vi "日志报警状态存储 (子VI).vi"() -> ()   [LabVIEW 2016, in "斯坦道CODMn.lvlib"]
uses:
  <vilib>/ptbypt/NI_PtbyPt.lvlib
  <vilib>/Utility/config.llb/NI_LVConfig.lvlib
panel:
  out "多列列表框":i32(listbox)
  out "CODMn工作状态":T1(ring)
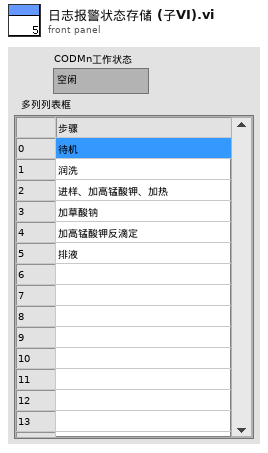
[diagram p1: front panel]
types:
  T1 = enum16{"空闲", "水样测试", "标样核查", "零点核查", "跨度核查", "空白测试", "平行样测试", "质控样", "空白校准", "标样校准", "加标回收"}
  T2 = cluster{"时间标识":timestamp, "设备":string, "日志信息":string}
  T3 = cluster{"时间标识":timestamp, "参数":string, "日志信息":string, "流程参数":string}
  T4 = cluster{"ORP故障":bool, "温控器故障":bool, "加热故障":bool, "高锰酸钾报警":bool, "草酸钠报警":bool, "测量错误":bool, "校零错误":bool, "校标错误":bool, " 进水样超量程":bool, "排液阀故障":bool, "60分钟超时报警":bool, "进样无液体报警":bool}
  T5 = cluster{"时间标识":timestamp, "设备":string, "日志信息":string, "流程参数":string}
  T6 = cluster{"测量量程":dbl, "测量精度":dbl, "测量间隔":dbl, "消解温度":dbl, "消解时长":dbl, "空白校准时间":timestamp, "曲线截距":dbl, "曲线斜率":dbl, "测量检出限":dbl, "测量信号值":dbl, "线性相关系数":dbl, "二次多项式系数":dbl, "标样校准时间":timestamp, "单位":u16}
  T7 = typedef "NI_LVConfig.lvlib/Config Data RefNum.ctl" = refnum<k1>
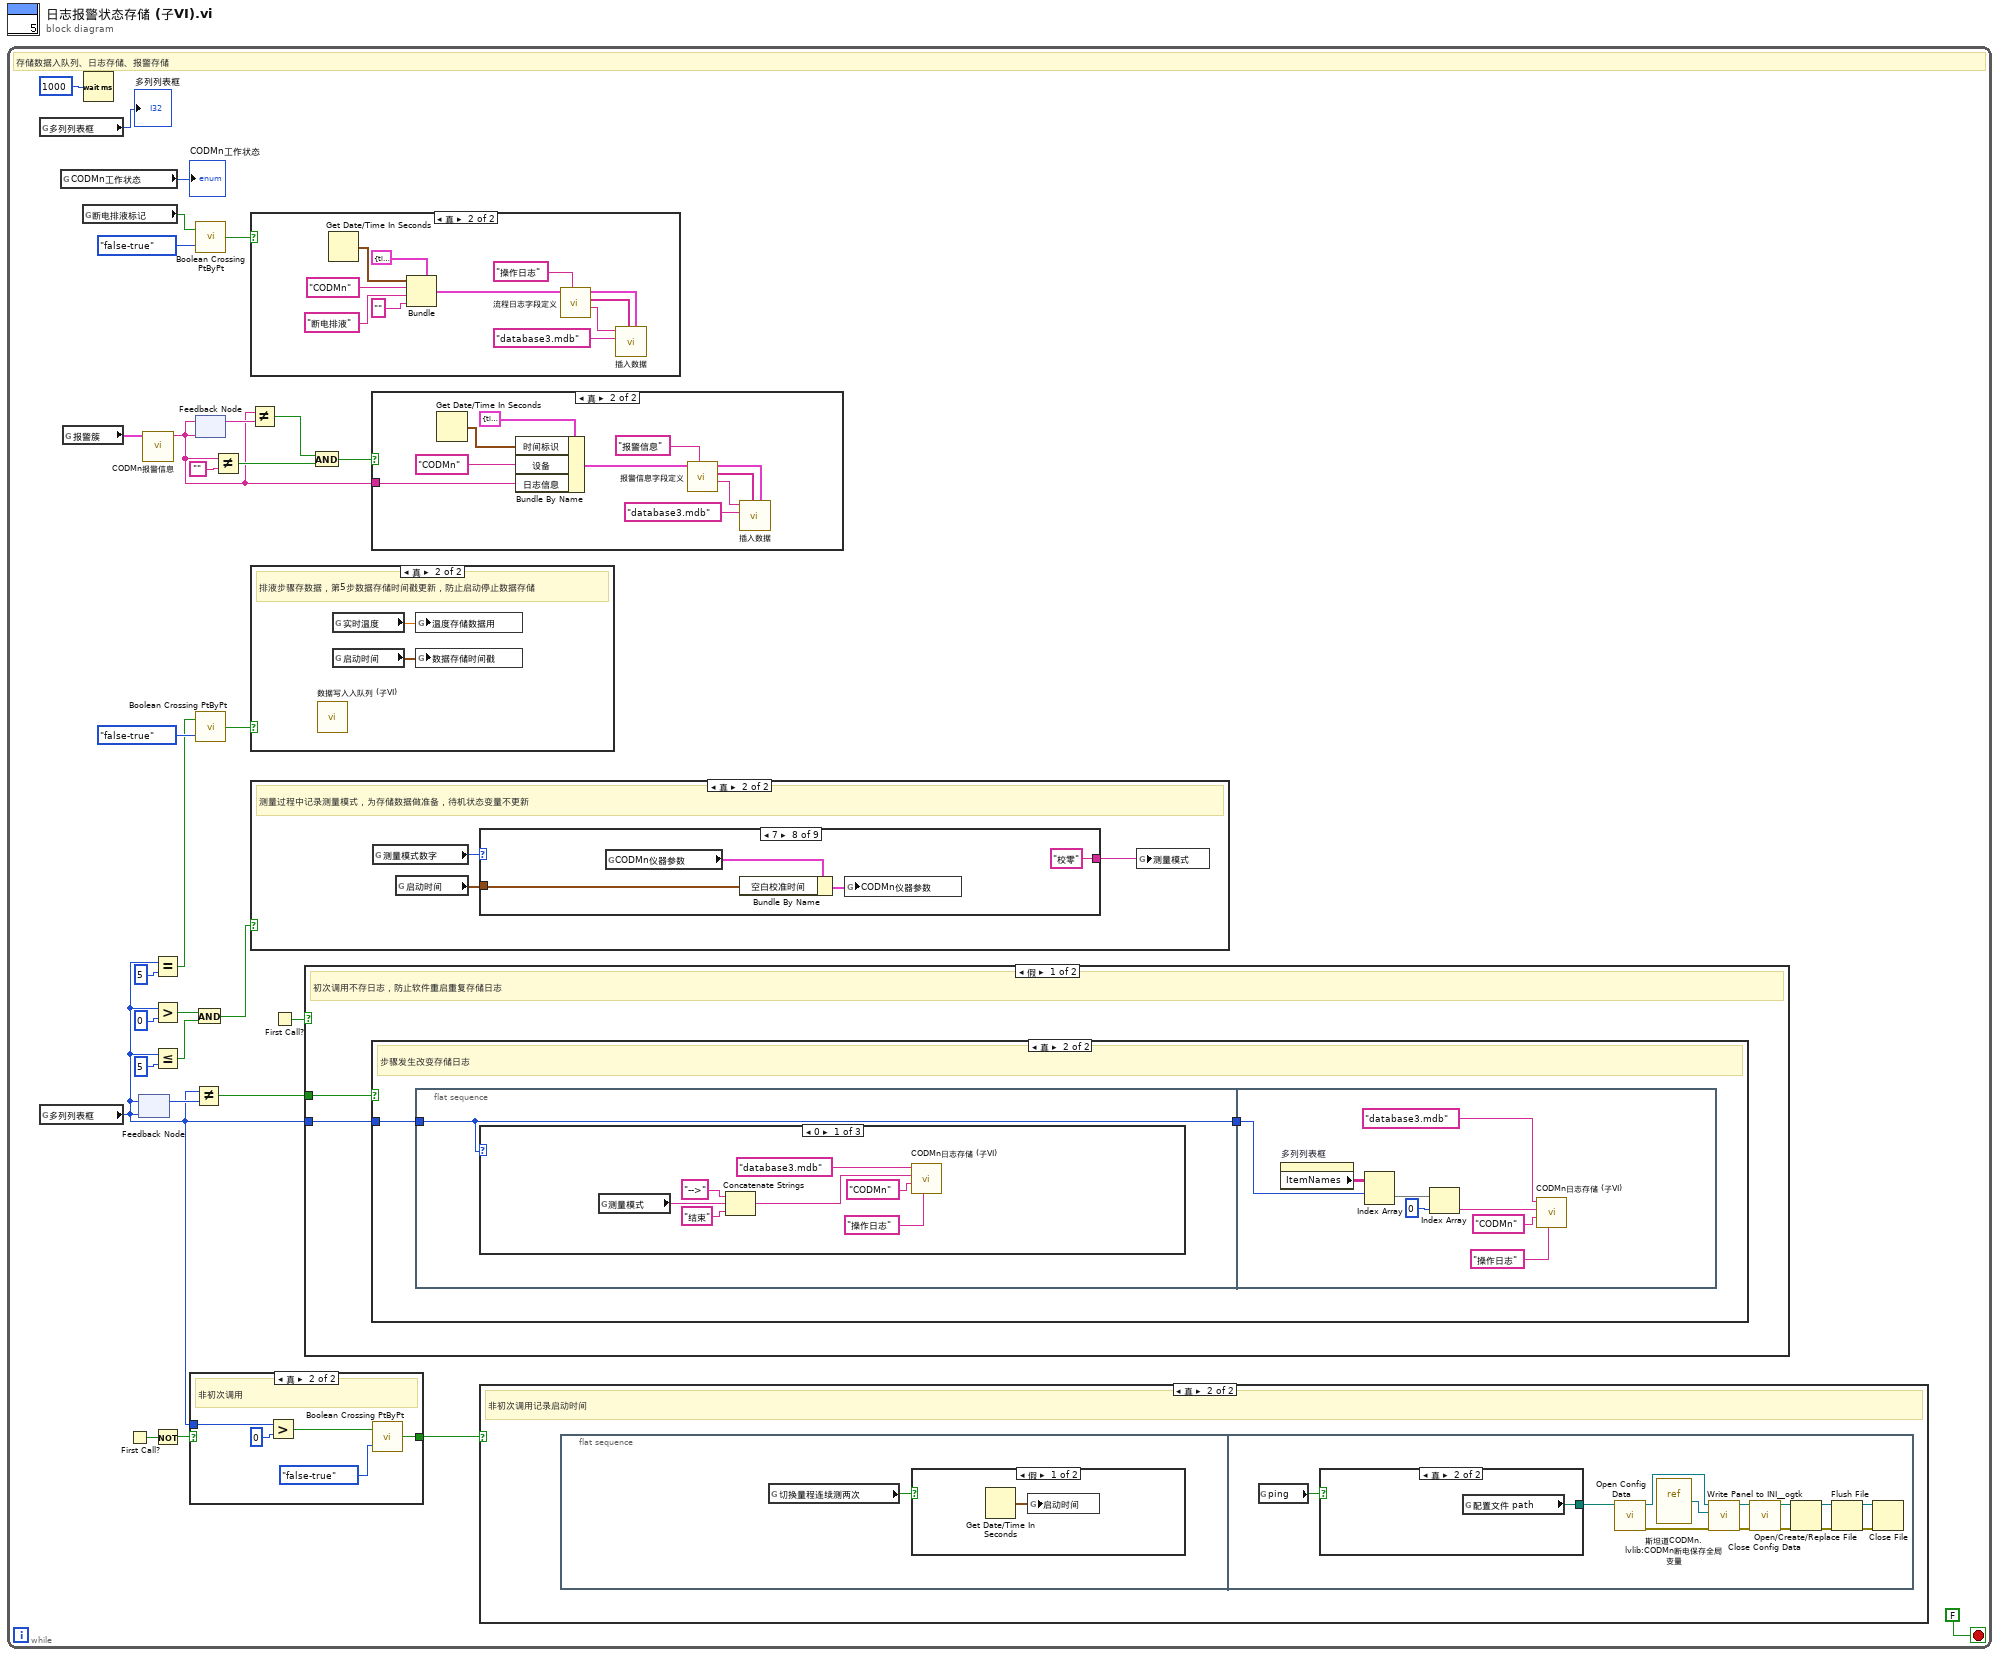
[diagram p0: block diagram]
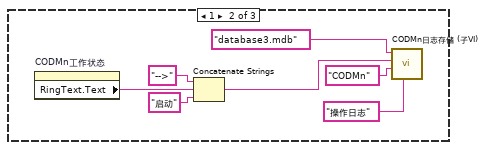
[diagram p3: hidden frame]
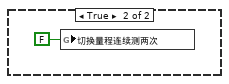
[diagram p10: hidden frame]
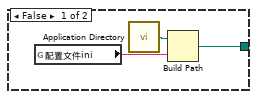
[diagram p11: hidden frame]
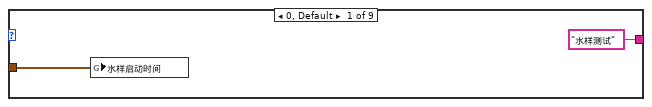
[diagram p13: hidden frame]
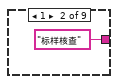
[diagram p14: hidden frame]
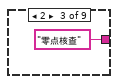
[diagram p15: hidden frame]
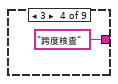
[diagram p16: hidden frame]
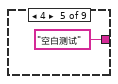
[diagram p17: hidden frame]
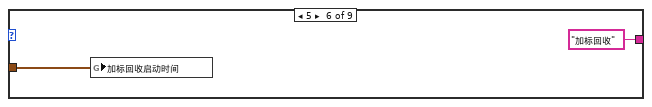
[diagram p18: hidden frame]
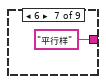
[diagram p19: hidden frame]
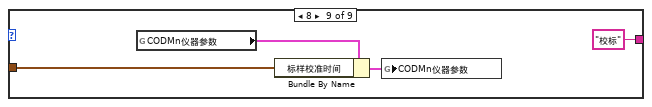
[diagram p20: hidden frame]
diagram:
  n1 = while {
    stop <- FALSE stop-if-true
    # "存储数据入队列、日志存储、报警存储"
    n2 = global read "运行时序全局变量.vi" "多列列表框"() -> (→"多列列表框":i32)
    n3 = global read "运行时序全局变量.vi" "多列列表框"() -> (w5:i32)
    n4 = global read "COD测量模式全局.vi" "CODMn工作状态"() -> (→"CODMn工作状态":T1)
    n5 = global read "COD内部交互全局.vi" "报警簇"() -> (w4:T4)
    n6 = global read "COD内部交互全局.vi" "断电排液标记"() -> (w3:bool)
    n7 = Wait (ms)(milliseconds to wait=u32 1000 ("等待时间（毫秒）")) -> ()  [unwired: 1 out]
    n8 = First Call?() -> (First Call?: T/F=w8:bool)
    n9 = feedback #1(w5) -> (w19:i32)
    n10 = feedback-in #1(w5) -> ()
    n11 = call "CODMn报警信息.vi"("报警簇"=w4) -> ("CODMN报警信息"=w9:string)  [unwired: 10 in]
    n12 = Equal?(x=w5, y=u16 5) -> (x = y?=w23:bool)
    n13 = Greater?(x=w5, y=u16 0) -> (0:w30:bool)
    n14 = Less Or Equal?(x=w5, y=u16 5) -> (x <= y?=w27:bool)
    n15 = Not(x=w8) -> (.not. x?=w6:bool)
    n16 = case shown="真" w6 {
      selector: w6 -> [w58 _]
      tunnel: w5 -> [_ w60]
      tunnel: [w58 w59] -> w7
      frame False {
      }
      frame True {
        # "非初次调用"
        n17 = Greater?(x=w60, y=u16 0) -> (0:w63:bool)
        n18 = call <vilib>:"Boolean Crossing PtByPt.vi"("direction"=enum16{"either", "false-true", "true-false"}."false-true", "input"=w63) -> ("crossing"=w59:bool)  [unwired: 1 in]
      }
    }
    n19 = Not Equal?(x=w5, y=w19) -> (x != y?=w20:bool)
    n20 = And(x=w30, y=w27) -> (x .and. y?=w28:bool)
    n21 = call <vilib>:"Boolean Crossing PtByPt.vi"("direction"=enum16{"either", "false-true", "true-false"}."false-true", "input"=w3) -> ("crossing"=w15:bool)  [unwired: 1 in]
    n22 = feedback #2(w9) -> (w10:string)
    n23 = feedback-in #2(w9) -> ()
    n24 = call <vilib>:"Boolean Crossing PtByPt.vi"("direction"=enum16{"either", "false-true", "true-false"}."false-true", "input"=w23) -> ("crossing"=w25:bool)  [unwired: 1 in]
    n25 = Not Equal?(x=w9, y="") -> (x != y?=w14:bool)
    n26 = Not Equal?(x=w9, y=w10) -> (x != y?=w11:bool)
    n27 = case shown="真" w15 {
      frame False {
      }
      frame True {
        n28 = Get Date/Time In Seconds() -> (seconds since 1Jan1904=w79:timestamp)
        n29 = Bundle(cluster=T3 {"时间标识"=timestamp(0 s since 1904-01-01), "参数"="", "日志信息"="", "流程参数"=""} ("data in"), "时间标识"=w79, "参数"="CODMn" ("table输入"), "日志信息"="断电排液", "流程参数"="" ("table输入")) -> (w77:T3)
        n30 = call "流程日志字段定义.vi"("table输入"="操作日志", "data in"=w77) -> ("table输出"=w82:string, "columns"=w83:string[], "data out"=w84:T5)  [unwired: 7 in]
        n31 = call "插入数据.vi"("data"=w84, "columns"=w83, "database"="database3.mdb", "table"=w82) -> ()  [unwired: 7 in, 1 out]
      }
    }
    n32 = case shown="真" w25 {
      frame False {
      }
      frame True {
        # "排液步骤存数据，第5步数据存储时间戳更新，防止启动停止数据存储"
        n33 = call "数据写入入队列 (子VI).vi"() -> ()  [unwired: 12 in]
        n34 = global read "COD内部交互全局.vi" "实时温度"() -> (w125:dbl)
        n35 = global read "CODMn断电保存全局变量.vi" "启动时间"() -> (w126:timestamp)
        n36 = global write "COD内部交互全局.vi" "温度存储数据用"(w125) -> ()
        n37 = global write "COD内部交互全局.vi" "数据存储时间戳"(w126) -> ()
      }
    }
    n38 = case shown="真" w28 {
      frame False {
      }
      frame True {
        # "测量过程中记录测量模式，为存储数据做准备，待机状态变量不更新"
        n39 = global read "COD内部交互全局.vi" "测量模式数字"() -> (w106:i32)
        n40 = global read "CODMn断电保存全局变量.vi" "启动时间"() -> (w105:timestamp)
        n41 = case shown="7" w106 {
          tunnel: ["水样测试" ("测量模式") "标样核查" ("测量模式") "零点核查" ("测量模式") "跨度核查" ("测量模式") "空白测试" ("测量模式") "加标回收" ("测量模式") "平行样" ("测量模式") "校零" ("测量模式") "校标" ("测量模式")] -> w107
          tunnel: w105 -> [w108 _ _ _ _ w114 _ w117 w121]
          frame 0, Default {
            n42 = global write "COD测量模式全局.vi" "水样启动时间"(w108) -> ()
          }
          frame 1 {
          }
          frame 2 {
          }
          frame 3 {
          }
          frame 4 {
          }
          frame 5 {
            n43 = global write "COD测量模式全局.vi" "加标回收启动时间"(w114) -> ()
          }
          frame 6 {
          }
          frame 7 {
            n44 = global read "CODMn断电保存全局变量.vi" "CODMn仪器参数"() -> (w119:T6)
            n45 = Bundle By Name(cluster=w119, "空白校准时间"=w117) -> (w118:T6)
            n46 = global write "CODMn断电保存全局变量.vi" "CODMn仪器参数"(w118) -> ()
          }
          frame 8 {
            n47 = global read "CODMn断电保存全局变量.vi" "CODMn仪器参数"() -> (w123:T6)
            n48 = Bundle By Name(cluster=w123, "标样校准时间"=w121) -> (w122:T6)
            n49 = global write "CODMn断电保存全局变量.vi" "CODMn仪器参数"(w122) -> ()
          }
        }
        n50 = global write "COD测量模式全局.vi" "测量模式"(w107) -> ()
      }
    }
    n51 = First Call?() -> (First Call?: T/F=w21:bool)
    n52 = case shown="假" w21 {
      tunnel: w20 -> [w32 _]
      tunnel: w5 -> [w31 _]
      frame False {
        # "初次调用不存日志，防止软件重启重复存储日志"
        n53 = case shown="真" w32 {
          tunnel: w31 -> [_ w34]
          frame False {
          }
          frame True {
            # "步骤发生改变存储日志"
            n54 = flat-sequence {
              tunnel: w34 -> [w35]
              tunnel: [w35] -> w33
              tunnel: w33 -> [w55]
              frame #0 {
                n55 = case shown="0" w35 {
                  frame 0 {
                    n56 = global read "COD测量模式全局.vi" "测量模式"() -> (w42:string)
                    n57 = Concatenate Strings("-->", w42, "结束" ("字符串")) -> (w41:string)
                    n58 = call "CODMn日志存储 (子VI).vi"("table输入"="操作日志", "参数"="CODMn" ("table输入"), "日志信息"=w41, "database"="database3.mdb") -> ()  [unwired: 8 in]
                  }
                  frame 1 {
                    n59 = property on="CODMn工作状态" class="Enum (严格)"() -> ("RingText.Text"=w43:string)  [unwired: 2 in, 2 out]
                    n60 = Concatenate Strings("-->", w43, "启动" ("字符串")) -> (w44:string)
                    n61 = call "CODMn日志存储 (子VI).vi"("table输入"="操作日志", "参数"="CODMn" ("table输入"), "日志信息"=w44, "database"="database3.mdb") -> ()  [unwired: 8 in]
                  }
                  frame 2, Default {
                  }
                }
              }
              frame #1 {
                n62 = property on="多列列表框" class="MCListbox (严格)"() -> ("ItemNames"=w50:string[][])  [unwired: 2 in, 2 out]
                n63 = Index Array(array=w50, index (row)=w55) -> (element=w53:string[])  [unwired: 1 in]
                n64 = Index Array(array=w53, index=0 ("索引")) -> (element=w51:string)
                n65 = call "CODMn日志存储 (子VI).vi"("table输入"="操作日志", "参数"="CODMn" ("table输入"), "日志信息"=w51, "database"="database3.mdb") -> ()  [unwired: 8 in]
              }
            }
          }
        }
      }
      frame True {
      }
    }
    n66 = And(x=w11, y=w14) -> (x .and. y?=w12:bool)
    n67 = case shown="真" w12 {
      tunnel: w9 -> [_ w64]
      frame False {
      }
      frame True {
        n68 = Get Date/Time In Seconds() -> (seconds since 1Jan1904=w66:timestamp)
        n69 = Bundle By Name(cluster=T2 {"时间标识"=timestamp(0 s since 1904-01-01), "设备"="", "日志信息"=""} ("data in"), "时间标识"=w66, "设备"="CODMn", "日志信息"=w64) -> (w67:T2)
        n70 = call "报警信息字段定义.vi"("table输入"="报警信息", "data in"=w67) -> ("table输出"=w71:string, "columns"=w72:string[], "data out"=w73:T2)  [unwired: 7 in]
        n71 = call "插入数据.vi"("data"=w73, "columns"=w72, "database"="database3.mdb", "table"=w71) -> ()  [unwired: 7 in, 1 out]
      }
    }
    n72 = case shown="真" w7 {
      frame False {
      }
      frame True {
        # "非初次调用记录启动时间"
        n73 = flat-sequence {
          frame #0 {
            n74 = global read "COD内部交互全局.vi" "切换量程连续测两次"() -> (w85:bool)
            n75 = case shown="假" w85 {
              frame False {
                n76 = Get Date/Time In Seconds() -> (seconds since 1Jan1904=w86:timestamp)
                n77 = global write "CODMn断电保存全局变量.vi" "启动时间"(w86) -> ()
              }
              frame True {
                n78 = global write "COD内部交互全局.vi" "切换量程连续测两次"(FALSE ("切换量程连续测两次")) -> ()
              }
            }
          }
          frame #1 {
            n79 = global read "CODMN外部API.vi" "ping"() -> (w89:bool)
            n80 = case shown="真" w89 {
              tunnel: [w101 w104] -> w88
              frame False {
                n81 = global read "COD内部交互全局.vi" "配置文件ini"() -> (w103:string)
                n82 = call <vilib>:"Application Directory.vi"() -> ("Application Directory"=w102:path)
                n83 = Build Path(base path=w102, name or relative path=w103) -> (appended path=w101:path)
              }
              frame True {
                n84 = global read "CODMN外部API.vi" "配置文件 path"() -> (w104:path)
              }
            }
            n85 = call <vilib>:"Open Config Data.vi"("configuration file path"=w88) -> ("error out"=w97:errorcluster, "refnum"=w100:T7)  [unwired: 8 in, 1 out]
            n86 = vi-ref "斯坦道CODMn.lvlib:CODMn断电保存全局变量.vi"() -> (w99:refnum<vi>)
            n87 = call <userlib>:"Write Panel to INI__ogtk.vi"("error in (no error)"=w97, "VI ref"=w99, "refnum"=w100) -> ("error out"=w96:errorcluster, "refnum out"=w98:T7)  [unwired: 7 in]
            n88 = call <vilib>:"Close Config Data.vi"("error in (no error)"=w96, "refnum"=w98) -> ("error out"=w91:errorcluster, "file path"=w90:path)  [unwired: 8 in]
            n89 = Open/Create/Replace File(file path (use dialog)=w90, error in=w91) -> (refnum out=w94:refnum<file>, error out=w95:errorcluster)  [unwired: 4 in, 1 out]
            n90 = Flush File(refnum=w94, error in=w95) -> (refnum out=w93:refnum<file>, error out=w92:errorcluster)
            n91 = Close File(refnum=w93, error in=w92) -> ()  [unwired: 2 out]
          }
        }
      }
    }
  }
